vi "create_reference_image.vi"(8 "error in (no error)":errorcluster, 11 "ColorOverlay in":refnum<class "ColorOverlay.lvclass">) -> (0 "error out":errorcluster, 2 "reference image out":T1(plugin-control), 3 "ColorOverlay out":refnum<class "ColorOverlay.lvclass">)   [LabVIEW 2010, in "ColorOverlay.lvclass"]
uses:
  ColorOverlay.lvclass
  ColorOverlay.lvclass/ColorOverlay.ctl
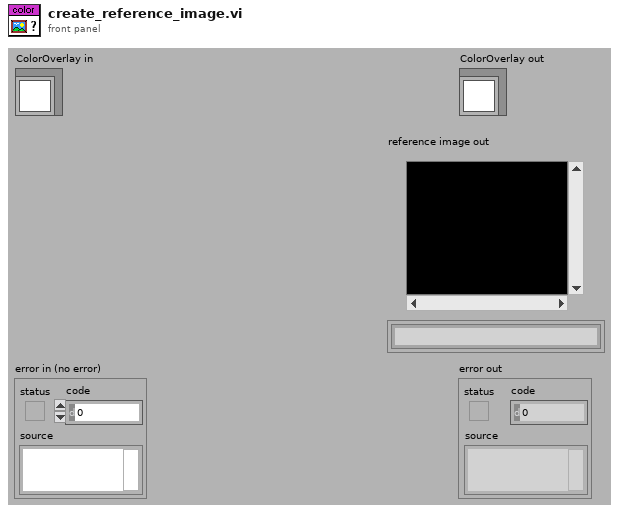
[diagram p1: front panel]
types:
  T1 = typedef "IMAQ Image.ctl" = refnum<image>
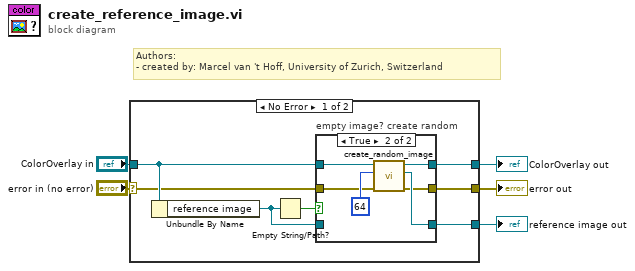
[diagram p0: block diagram]
diagram:
  # "Authors: \n- created by: Marcel van 't Hoff, University of Zurich, Switzerland"
  n1 = case shown="No Error" "error in (no error)" {
    selector: "error in (no error)" -> [w7 w23]
    tunnel: [w6 w23] -> w4
    tunnel: [w11 w22] -> w2
    tunnel: "ColorOverlay in" -> [w12 w22]
    tunnel: [w9 _] -> w1
    frame No Error {
      n2 = Unbundle By Name(w12) -> ("reference image"=w8:T1)
      n3 = Empty String/Path?(string/path=w8) -> (empty?=w10:bool)
      n4 = case "empty image? create random" shown="True" w10 {
        tunnel: w12 -> [w13 w20]
        tunnel: [w13 w19] -> w11
        tunnel: [w15 w18] -> w9
        tunnel: w8 -> [w15 _]
        tunnel: w7 -> [w14 w17]
        tunnel: [w14 w16] -> w6
        frame False {
        }
        frame True {
          n5 = call-dynamic "create_random_image.vi"("error in (no error)"=w17, "array size"=64, "ColorOverlay in"=w20) -> ("error out"=w16:errorcluster, "random image out"=w18:T1, "ColorOverlay out"=w19:refnum<class "ColorOverlay.lvclass">)  [unwired: 6 in]
        }
      }
    }
    frame Error {
    }
  }
  "error out" <- w4
  "ColorOverlay out" <- w2
  "reference image out" <- w1
